vi "SUBVI_MDT693B_write.vi"(7 "z":dbl, 8 "error in (no error)":errorcluster, 9 "y":dbl, 10 "x":dbl, 11 "VISA Refnum in":refnum<visa-resource-name>) -> (0 "error out":errorcluster, 3 "VISA Refnum out":refnum<visa-resource-name>)   [LabVIEW 2020]
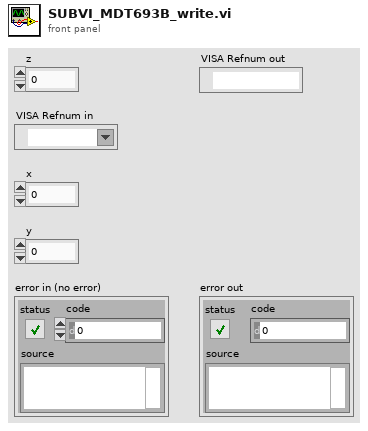
[diagram p1: front panel]
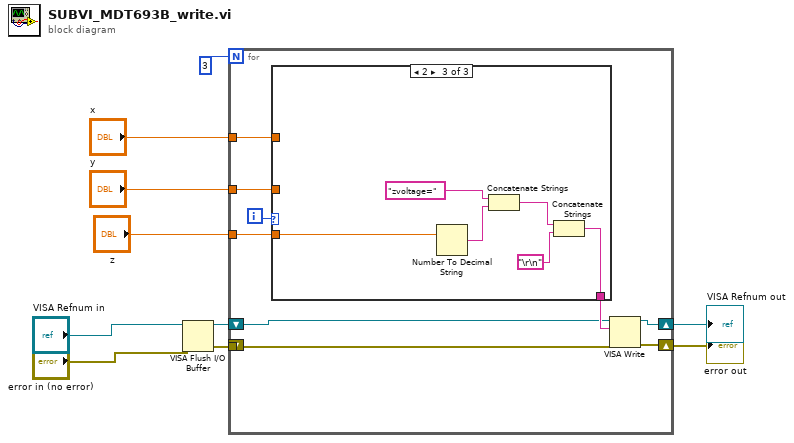
[diagram p0: block diagram]
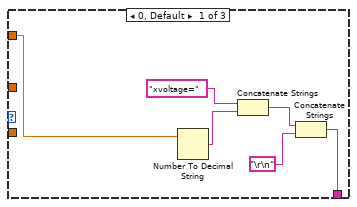
[diagram p2: hidden frame]
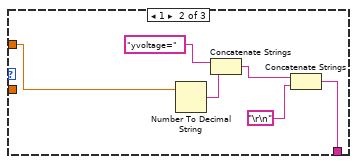
[diagram p3: hidden frame]
diagram:
  n1 = VISA Flush I/O Buffer(VISA resource name="VISA Refnum in", error in (no error)="error in (no error)") -> (VISA resource name out=w7:refnum<visa-resource-name>, error out=w6:errorcluster)  [unwired: 1 in]
  n2 = for {
    N: 3 -> [_]
    tunnel: w6 -> [w16]
    shift-right: [w15] -> w2
    shift-left: _ -> [_]
    shift-right: [w14] -> w3
    shift-left: w7 -> [w17]
    tunnel: "x" -> [w13]
    tunnel: "y" -> [w12]
    tunnel: "z" -> [w11]
    i -> [w19]
    n3 = case shown="2" w19 {
      tunnel: [w21 w27 w33] -> w18
      tunnel: w13 -> [w20 _ _]
      tunnel: w12 -> [_ w26 _]
      tunnel: w11 -> [_ _ w32]
      frame 0, Default {
        n4 = Number To Decimal String(number=w20) -> (decimal integer string=w24:string)  [unwired: 1 in]
        n5 = Concatenate Strings("xvoltage=", w24) -> (w23:string)
        n6 = Concatenate Strings(w23, "\r\n") -> (w21:string)
      }
      frame 1 {
        n7 = Number To Decimal String(number=w26) -> (decimal integer string=w30:string)  [unwired: 1 in]
        n8 = Concatenate Strings("yvoltage=", w30) -> (w29:string)
        n9 = Concatenate Strings(w29, "\r\n") -> (w27:string)
      }
      frame 2 {
        n10 = Number To Decimal String(number=w32) -> (decimal integer string=w34:string)  [unwired: 1 in]
        n11 = Concatenate Strings("zvoltage=", w34) -> (w36:string)
        n12 = Concatenate Strings(w36, "\r\n") -> (w33:string)
      }
    }
    n13 = VISA Write(VISA resource name=w17, write buffer=w18, error in (no error)=w16) -> (VISA resource name out=w14:refnum<visa-resource-name>, error out=w15:errorcluster)  [unwired: 1 out]
  }
  "VISA Refnum out" <- w3
  "error out" <- w2
